vi "UR Server.vi"() -> ()   [LabVIEW 2016]
panel:
  out "size(s)":i32
  out "data":string
  out "connected":bool
  in  "stop":bool
  in  "rcv":bool
  out "data out":string
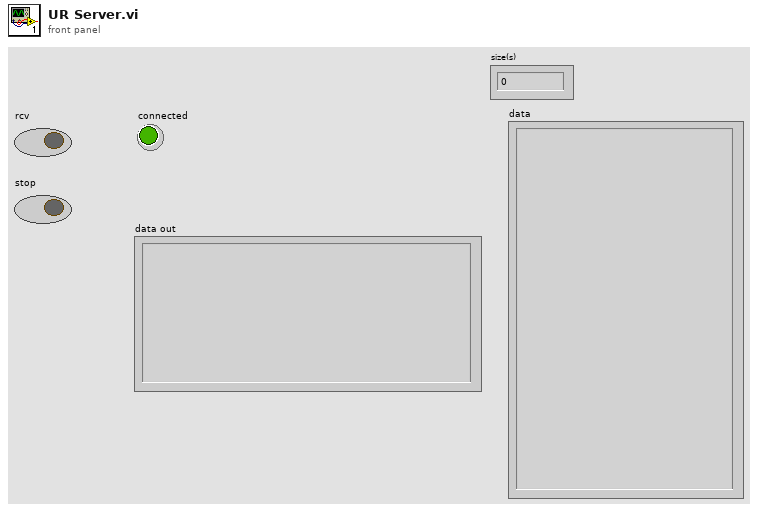
[diagram p1: front panel]
types:
  T1 = enum16{"Standard", "Buffered", "CRLF", "Immediate"}
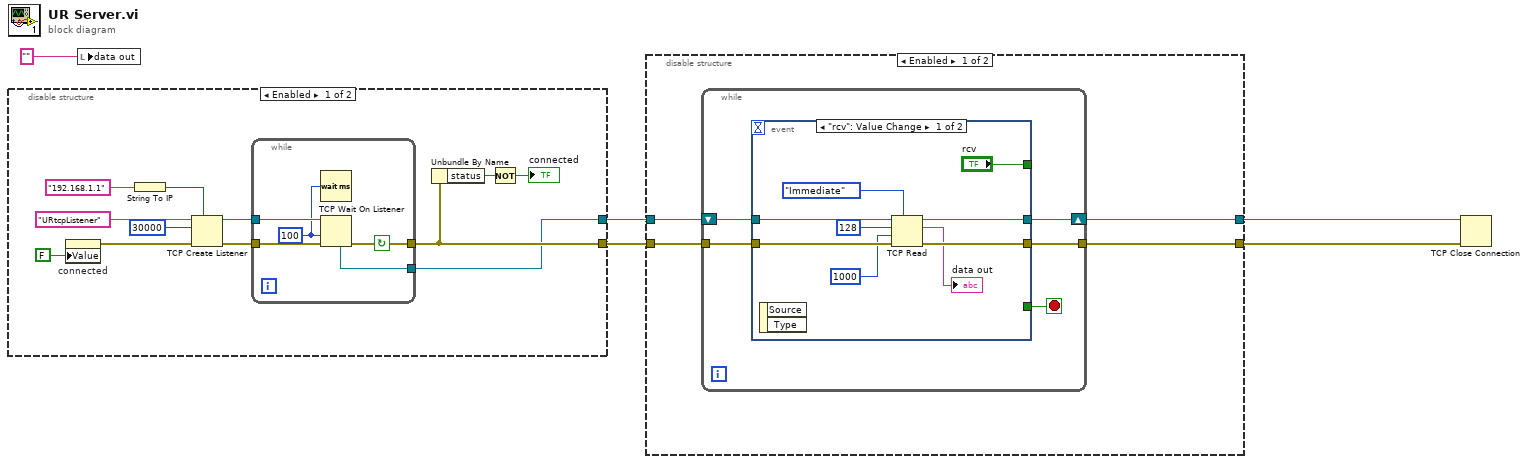
[diagram p0: block diagram]
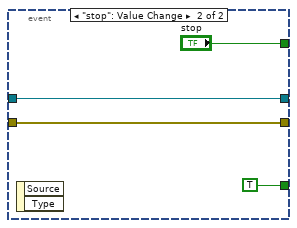
[diagram p2: hidden frame]
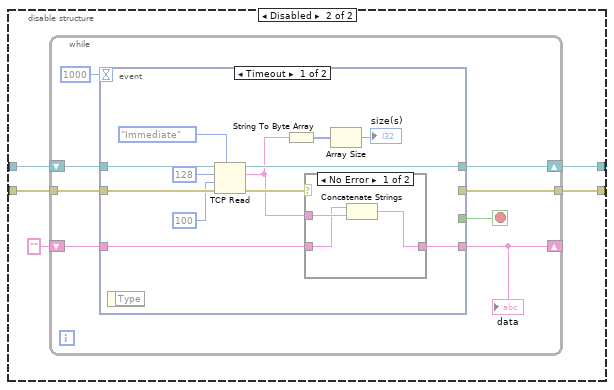
[diagram p3: hidden frame]
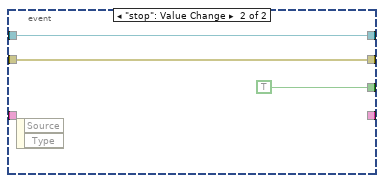
[diagram p5: hidden frame]
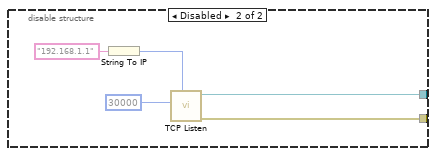
[diagram p6: hidden frame]
diagram:
  n1 = disable-structure shown="Enabled" {
    disable-tunnel: [w6 w24] -> w3
    disable-tunnel: [w11 w23] -> w2
    frame Enabled {
      n2 = property on="connected" class="Bool (strict)"("Value"=FALSE ("connected")) -> (error out=w8:errorcluster)  [unwired: 2 in, 1 out]
      n3 = String To IP(1:"192.168.1.1" ("name")) -> (0:w15:u32)
      n4 = TCP Create Listener(7:w15, 8:w8, 10:u16 30000 ("remote port or service name"), 11:"URtcpListener" ("service name")) -> (0:w12:errorcluster, 3:w13:refnum<k5>)  [unwired: 1 in, 1 out]
      n5 = while {
        tunnel: w12 -> [w21]
        tunnel: [w19] -> w11
        tunnel: [w18] -> w6
        tunnel: w13 -> [w22]
        stop <- w19 continue-if-true
        w20 = 100 ("timeout ms (wait forever: -1)")
        n6 = Wait (ms)(milliseconds to wait=w20) -> ()  [unwired: 1 out]
        n7 = TCP Wait On Listener(8:w21, 9:w20, 11:w22) -> (0:w19:errorcluster, 4:w18:refnum<k5>)  [unwired: 1 in, 3 out]
      }
      n8 = Unbundle By Name(w11) -> ("status"=w10:bool)
      n9 = Not(x=w10) -> (.not. x?=→"connected":bool)
    }
    frame Disabled {
      n10 = String To IP(1:"192.168.1.1" ("name")) -> (0:w26:u32)
      n11 = call <vilib>:"TCP Listen.vi"("net address"=w26, "port"=u16 30000 ("remote port or service name")) -> ("error out"=w23:errorcluster, "connection ID"=w24:refnum<k5>)  [unwired: 5 in, 3 out]
    }
  }
  n12 = local write "data out"("" ("data out")) -> ()
  n13 = disable-structure shown="Enabled" {
    disable-tunnel: [w31 w54] -> w5
    disable-tunnel: [w30 w53] -> w4
    disable-tunnel: w3 -> [w29 w52]
    disable-tunnel: w2 -> [w28 w51]
    frame Enabled {
      n14 = while {
        shift-right: [w36] -> w31
        shift-left: w29 -> [w33]
        tunnel: w28 -> [w34]
        tunnel: [w35] -> w30
        stop <- w32 stop-if-true
        n15 = event shown="[0] \"rcv\": Value Change" {
          selector: _ -> [_ _]
          dyn-events: _ -> [_ _]
          timeout: _ -> [_ _]
          tunnel: [w45 w48] -> w36
          tunnel: [w44 w47] -> w35
          tunnel: w34 -> [w43 w47]
          tunnel: w33 -> [w42 w48]
          tunnel: ["rcv" "stop"] -> _
          tunnel: [_ TRUE] -> w32
          event "rcv": Value Change {
            n16 = event-data() -> ()  [unwired: 1 in, 2 out]
            n17 = TCP Read(connection ID=w42, bytes to read=128, error in (no error)=w43, 7:T1."Immediate" ("mode (standard)"), 9:1000 ("timeout ms (25000)")) -> (connection ID out=w45:refnum<k5>, data out=→"data out":string, error out=w44:errorcluster)
          }
          event "stop": Value Change {
            n18 = event-data() -> ()  [unwired: 1 in, 2 out]
          }
        }
      }
    }
    frame Disabled {
      n19 = while {
        shift-right: [w62] -> w54
        shift-left: w52 -> [w59]
        tunnel: w51 -> [w60]
        tunnel: [w61] -> w53
        shift-right: [w56] -> _
        shift-left: "" -> [w55]
        stop <- w58 stop-if-true
        n20 = event shown="[0] Timeout" {
          selector: _ -> [_ _]
          dyn-events: _ -> [_ _]
          timeout: 1000 -> [_ _]
          tunnel: [w74 w81] -> w62
          tunnel: [_ w80] -> w61
          tunnel: w60 -> [w73 w80]
          tunnel: w59 -> [w72 w81]
          tunnel: [_ TRUE] -> w58
          tunnel: [w70 _] -> w56
          tunnel: w55 -> [w69 _]
          event Timeout {
            n21 = event-data() -> ()  [unwired: 1 in, 1 out]
            n22 = TCP Read(connection ID=w72, bytes to read=128, error in (no error)=w73, 7:T1."Immediate" ("mode (standard)"), 9:100 ("timeout ms (25000)")) -> (connection ID out=w74:refnum<k5>, data out=w65:string, error out=w71:errorcluster)
            n23 = String To Byte Array(string=w65) -> (unsigned byte array=w64:u8[])
            n24 = case shown="No Error" w71 {
              tunnel: w65 -> [w77 _]
              tunnel: [w76 w78] -> w70
              tunnel: w69 -> [w75 w78]
              frame No Error {
                n25 = Concatenate Strings(w75, w77) -> (w76:string)
              }
              frame Error {
              }
            }
            n26 = Array Size(array=w64) -> (size(s)=→"size(s)":i32)
          }
          event "stop": Value Change {
            n27 = event-data() -> ()  [unwired: 1 in, 2 out]
          }
        }
        "data" <- w56
      }
    }
  }
  n28 = TCP Close Connection(connection ID=w5, error in (no error)=w4) -> ()  [unwired: 1 in, 2 out]
